vi "Z-Scan_acquisition.vi"() -> ()   [LabVIEW 2010]
uses:
  <vilib>/DAQmx/create/channels.llb/DAQmx Create Channel (AI-Voltage-Basic).vi
  <vilib>/DAQmx/configure/timing.llb/DAQmx Timing (Sample Clock).vi
  <vilib>/DAQmx/configure/trigger.llb/DAQmx Start Trigger (Digital Edge).vi
  <vilib>/Utility/file.llb/Write To Spreadsheet File (DBL).vi
  Arquivos de programas/National Instruments/LabVIEW 2010/resource/objmgr/daqmx.rc
panel:
  in  "lower threshold":dbl
  out "Ioca":cluster{dbl[], dbl[]}(graph)
  out "Ica":cluster{dbl[], dbl[]}(graph)
  in  "upper threshold":dbl
  out "Ioa":cluster{dbl[], dbl[]}(graph)
  in  "x step (mm)":dbl=5.0
  in  "x max (mm)":dbl=500.0
  in  "x min (mm)":dbl=-0.5
  in  "stop 10":bool
  in  "N":i32=1000
  in  "input terminal configuration":i32(ring)=10078 items=["default"=-1, "RSE"=10083, "NRSE"=10078, "Differential"=10106, "Pseudodifferential"=12529]
  in  "Signal":tag="Dev2/ai0"
  in  "Minimum value":dbl=-5.0
  in  "Maximum value":dbl=10.0
  in  "error array in":errorcluster[](array[cluster])
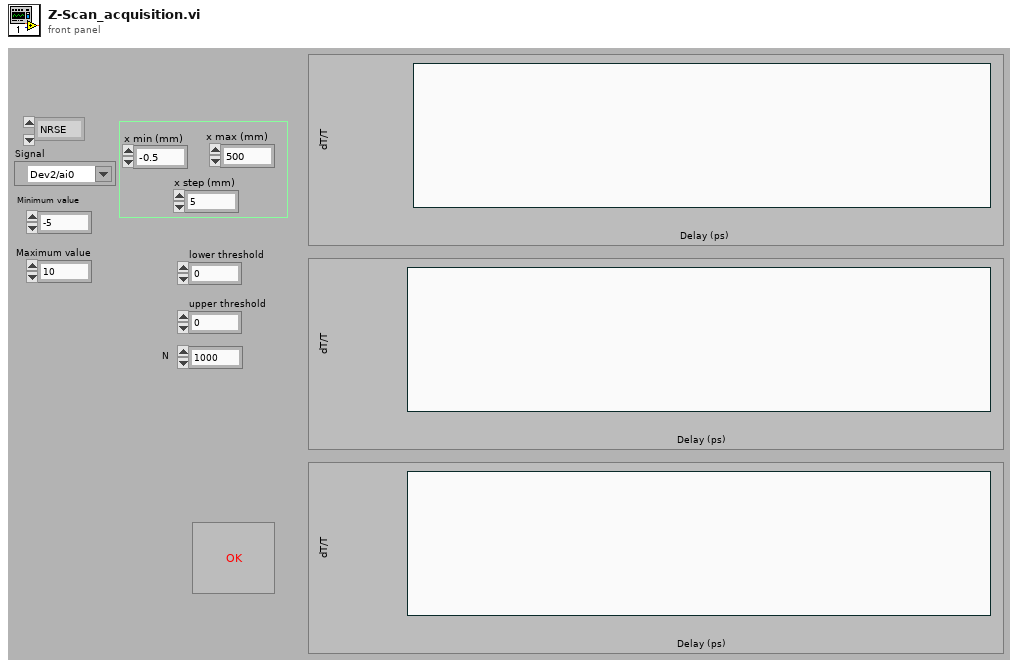
[diagram p1: front panel]
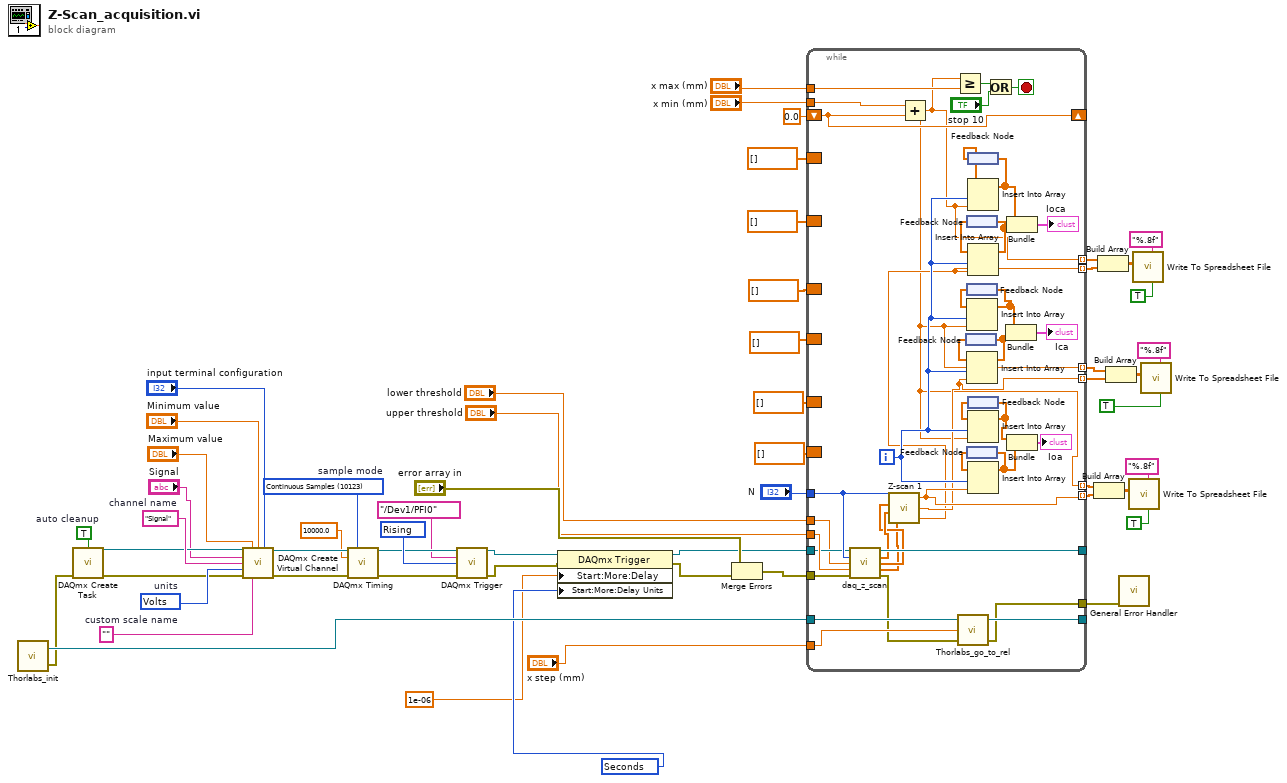
[diagram p0: block diagram]
diagram:
  w6 = 10364 items=["Sample Clock Periods"=10286, "Seconds"=10364, "Ticks"=10304] ("Start.DelayUnits")
  w48 = 10280 items=["Rising"=10280, "Falling"=10171] ("Trigger edge")
  w46 = 10123 items=["Finite Samples"=10178, "Continuous Samples"=10123, "Hardware Timed Single Point"=12522]  # sample mode
  w55 = 10348 items=["Volts"=10348, "From Custom Scale"=10065]  # units
  w54 = "Signal"  # channel name
  w56 = ""  # custom scale name
  w53 = TRUE  # auto cleanup
  n1 = call <userlib>:"Thorlabs_init.vi"() -> ("error out"=w7:errorcluster, "reference out"=w57:refnum<k7>)  [unwired: 2 in]
  n2 = call <vilib>:"DAQmx Create Task.vi"("auto cleanup"=w53, "error in"=w7) -> ("task out"=w52:refnum<k21>, "error out"=w50:errorcluster)  [unwired: 12 in]
  n3 = call-poly <vilib>:"DAQmx Create Virtual Channel.vi"("task in"=w52, "maximum value"="Maximum value", "minimum value"="Minimum value", "input terminal configuration"="input terminal configuration", "physical channels"="Signal", "name to assign"=w54, "units"=w55, "error in"=w50, "custom scale name"=w56) -> ("task out"=w40:refnum<k21>, "error out"=w39:errorcluster)  [unwired: 5 in]
  n4 = call-poly <vilib>:"DAQmx Timing.vi"("task/channels in"=w40, "sample mode"=w46, "rate"=10000.0, "error in"=w39) -> ("task out"=w47:refnum<k21>, "error out"=w44:errorcluster)  [unwired: 10 in]
  n5 = call-poly <vilib>:"DAQmx Trigger.vi"("task/channels in"=w47, "source"=tag "/Dev1/PFI0", "edge"=w48, "error in"=w44) -> ("task out"=w5:refnum<k21>, "error out"=w2:errorcluster)  [unwired: 10 in]
  n6 = property class="DAQmx Trigger"(reference=w5, error in=w2, "Start:More:Delay"=1e-06 ("Trigger Delay"), "Start:More:Delay Units"=w6) -> (reference out=w4:refnum<k21>, error out=w3:errorcluster)
  n7 = Merge Errors("error array in", w3) -> (w24:errorcluster)
  n8 = while {
    tunnel: "x max (mm)" -> [w92]
    tunnel: [w62] -> w33 mode=indexing
    tunnel: [w84] -> w32 mode=indexing
    tunnel: [w58] -> w25
    tunnel: [w86] -> _
    tunnel: "x min (mm)" -> [w87]
    tunnel: "x step (mm)" -> [w79]
    tunnel: w57 -> [w83]
    tunnel: [w88] -> _
    tunnel: "N" -> [w85]
    shift-right: [w80] -> _
    shift-left: 0.0 -> [w80]
    border: dbl[] [] -> [_]
    border: dbl[] [] -> [_]
    tunnel: w24 -> [w60]
    tunnel: "upper threshold" -> [w82]
    tunnel: w4 -> [w81]
    border: dbl[] [] -> [_]
    border: dbl[] [] -> [_]
    border: dbl[] [] -> [_]
    border: dbl[] [] -> [_]
    tunnel: [w64] -> w12 mode=indexing
    tunnel: [w62] -> w11 mode=indexing
    tunnel: [w63] -> w10 mode=indexing
    tunnel: [w62] -> w9 mode=indexing
    tunnel: "lower threshold" -> [w61]
    i -> [w68]
    stop <- w90 stop-if-true
    n9 = call <userlib>:"daq_z_scan.vi"("channels in"=w81, "N"=w85, "lower threshold"=w61, "upper threshold"=w82, "error in"=w60) -> ("task out"=w86:refnum<k21>, "CA"=w78:dbl[], "OA"=w77:dbl[], "Ref"=w76:dbl[], "error out"=w59:errorcluster)  [unwired: 6 in]
    n10 = call <userlib>:"Z-scan 1.vi"("Ref"=w76, "CA"=w78, "OA"=w77, "N"=w85) -> ("Ioca"=w63:dbl, "Ica"=w64:dbl, "Ioa"=w84:dbl)
    n11 = Add(x=w87, y=w80) -> (x+y=w62:dbl)
    n12 = Greater Or Equal?(x=w62, y=w92) -> (x >= y?=w91:bool)
    n13 = call <userlib>:"Thorlabs_go_to_rel.vi"("error in (no error)"=w59, "Step (mm)"=w79, "MG17Motor in"=w83) -> ("error out"=w58:errorcluster, "MG17Motor out"=w88:refnum<k7>)  [unwired: 1 out]
    n14 = feedback #1() -> (w75:dbl[])
    n15 = feedback #2() -> (w66:dbl[])
    n16 = feedback #3() -> (w72:dbl[])
    n17 = Insert Into Array(array=w72, index=w68, new element=w62) -> (w73:dbl[])
    n18 = feedback-in #3(w73) -> ()
    n19 = Insert Into Array(array=w75, index=w68, new element=w64) -> (w74:dbl[])
    n20 = feedback-in #1(w74) -> ()
    n21 = feedback #4() -> (w95:dbl[])
    n22 = feedback #5() -> (w67:dbl[])
    n23 = Insert Into Array(array=w67, index=w68, new element=w62) -> (w69:dbl[])
    n24 = feedback-in #5(w69) -> ()
    n25 = Insert Into Array(array=w66, index=w68, new element=w63) -> (w70:dbl[])
    n26 = feedback-in #2(w70) -> ()
    n27 = feedback #6() -> (w96:dbl[])
    n28 = Insert Into Array(array=w96, index=w68, new element=w62) -> (w93:dbl[])
    n29 = feedback-in #6(w93) -> ()
    n30 = Insert Into Array(array=w95, index=w68, new element=w84) -> (w94:dbl[])
    n31 = feedback-in #4(w94) -> ()
    n32 = Or(x=w91, y="stop 10") -> (x .or. y?=w90:bool)
    n33 = Bundle(w73, w74) -> (→"Ica":cluster{dbl[], dbl[]})  [unwired: 1 in]
    n34 = Bundle(w69, w70) -> (→"Ioca":cluster{dbl[], dbl[]})  [unwired: 1 in]
    n35 = Bundle(w93, w94) -> (→"Ioa":cluster{dbl[], dbl[]})  [unwired: 1 in]
  }
  n36 = Build Array(w33, w32) -> (w29:dbl[][])
  n37 = Build Array(w9, w10) -> (w13:dbl[][])
  n38 = Build Array(w11, w12) -> (w16:dbl[][])
  n39 = call <vilib>:"General Error Handler.vi"("error in (no error)"=w25) -> ()  [unwired: 10 in, 5 out]
  n40 = call-poly <vilib>:"Write To Spreadsheet File.vi"("transpose? (no:F)"=TRUE, "format (%.3f)"="%.8f", "2D data"=w29) -> ()  [unwired: 5 in, 1 out]
  n41 = call-poly <vilib>:"Write To Spreadsheet File.vi"("transpose? (no:F)"=TRUE, "format (%.3f)"="%.8f", "2D data"=w13) -> ()  [unwired: 5 in, 1 out]
  n42 = call-poly <vilib>:"Write To Spreadsheet File.vi"("transpose? (no:F)"=TRUE, "format (%.3f)"="%.8f", "2D data"=w16) -> ()  [unwired: 5 in, 1 out]
